vi "Thermal Chamber Response Simulator_Init.vi"(8 "error in (no error)":errorcluster) -> (0 "error out":errorcluster)   [LabVIEW 2018]
uses:
  <vilib>/addons/_JKI Toolkits/Caraya/classes/Test/Test.lvclass
  <vilib>/addons/_JKI Toolkits/Caraya/classes/Assert/Assert.lvclass
  Libraries/Thermal Chamber Response Simulator/Thermal Chamber Response Simulator.lvlib
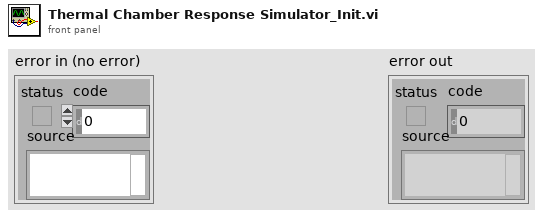
[diagram p1: front panel]
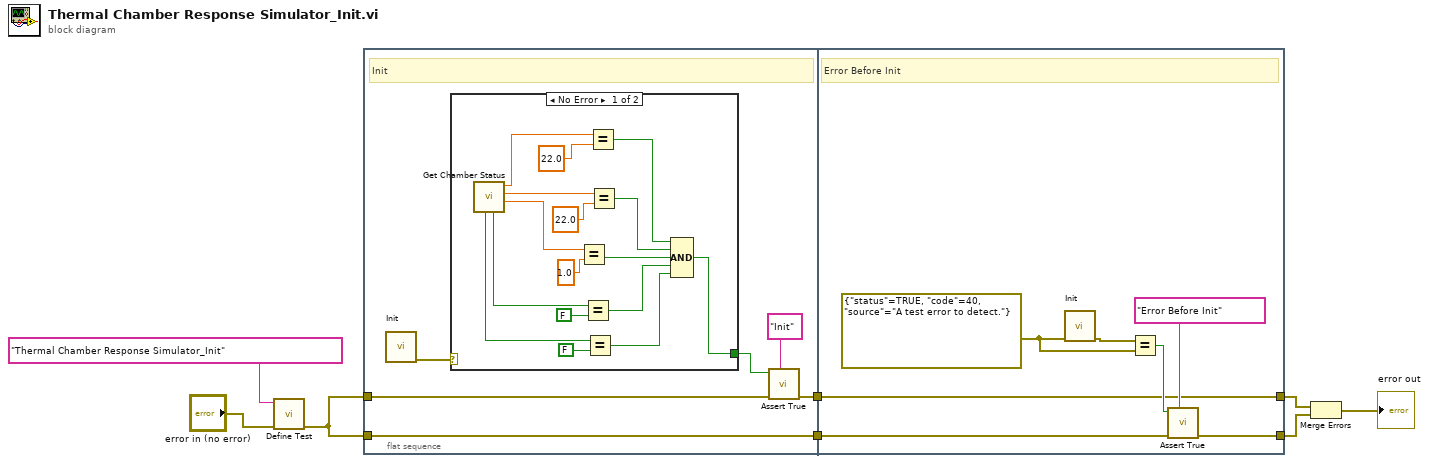
[diagram p0: block diagram]
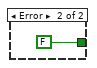
[diagram p2: hidden frame]
diagram:
  n1 = call <vilib>:"Define Test.vi"("error in (no error)"="error in (no error)", "Label (VI Title)"="Thermal Chamber Response Simulator_Init") -> ("error out"=w6:errorcluster)  [unwired: 9 in]
  n2 = flat-sequence {
    tunnel: w6 -> [w11]
    tunnel: [w10] -> w7
    tunnel: w6 -> [w9]
    tunnel: [w9] -> w5
    tunnel: [w35] -> w3
    tunnel: w7 -> [w34]
    tunnel: [w34] -> w4
    tunnel: w5 -> [w33]
    frame #0 {
      # "Init"
      n3 = call "Init.vi"() -> ("error out"=w14:errorcluster)  [unwired: 11 in]
      n4 = case shown="No Error" w14 {
        tunnel: [w15 FALSE] -> w12
        frame No Error {
          n5 = call "Get Chamber Status.vi"() -> ("Ramp Rate (deg C / second)"=w28:dbl, "Temperature Set Point (deg C)"=w29:dbl, "Actual Temperature"=w30:dbl, "Application Exit"=w27:bool, "Heater State"=w26:bool)  [unwired: 6 in, 1 out]
          n6 = Equal?(x=w28, y=1.0) -> (x = y?=w18:bool)
          n7 = Equal?(x=w27, y=FALSE) -> (x = y?=w17:bool)
          n8 = Equal?(x=w26, y=FALSE) -> (x = y?=w16:bool)
          n9 = Equal?(x=w30, y=22.0) -> (x = y?=w20:bool)
          n10 = Equal?(x=w29, y=22.0) -> (x = y?=w19:bool)
          n11 = Compound Arithmetic op=AND(w20, w19, w18, w17, w16) -> (w15:bool)
        }
        frame Error {
        }
      }
      n12 = call <vilib>:"Assert True.vi"("Label"="Init", "error in (no error)"=w11, "True?"=w12) -> ("error out"=w10:errorcluster)  [unwired: 8 in]
    }
    frame #1 {
      w32 = errorcluster {"status"=TRUE, "code"=40, "source"="A test error to detect."} ("Test Error")
      # "Error Before Init"
      n13 = call "Init.vi"("error in (no error)"=w32) -> ("error out"=w36:errorcluster)  [unwired: 10 in]
      n14 = Equal?(x=w36, y=w32) -> (x = y?=w37:bool)
      n15 = call <vilib>:"Assert True.vi"("Label"="Error Before Init", "error in (no error)"=w33, "True?"=w37) -> ("error out"=w35:errorcluster)  [unwired: 8 in]
    }
  }
  n16 = Merge Errors(w4, w3) -> (→"error out":errorcluster)
